vi "XCP DAQ Clear.vi"(8 "error in (no error)":errorcluster, 11 "DAQList in":refnum<class "DAQList.lvclass">) -> (0 "error out":errorcluster, 2 "ECU ref out":T1)   [LabVIEW 2019, in "XCP_DaqDtoId.lvlib" / "DAQList.lvclass"]
uses:
  DAQList.lvclass
  <vilib>/ECUMC/ECUMC.llb/MC Reference.ctt
  DAQList.lvclass/DAQList.ctl
  <vilib>/xnet/xnet.llb/XNET Control Scope.ctl
  <vilib>/ECUMC/ECUMC.lvlib
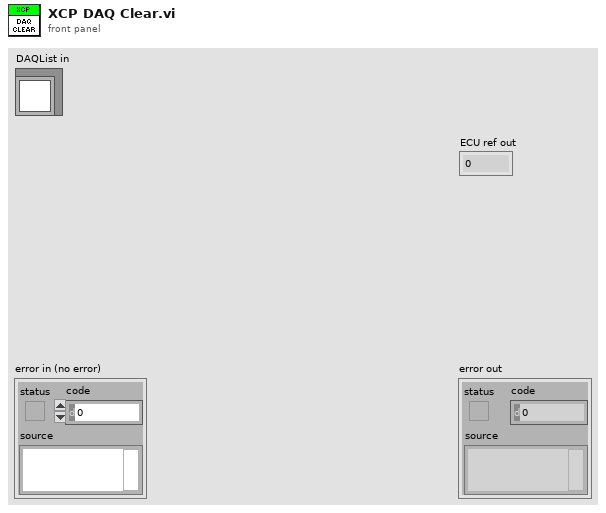
[diagram p1: front panel]
types:
  T1 = typedef "ECUMC.lvlib/MC Reference.ctt" = u32
  T2 = typedef "XNET Control Scope.ctl" = u32
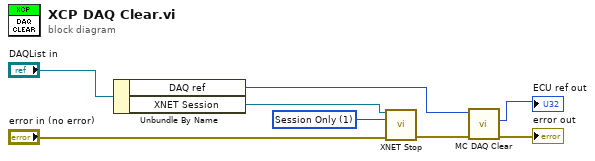
[diagram p0: block diagram]
diagram:
  w3 = T2 1 items=["Normal", "Session Only", "Interface Only", "Session Only Blocking"] ("scope (normal)")
  n1 = Unbundle By Name("DAQList in") -> ("DAQ ref"=w2:T1, "XNET Session"=w4:refnum<k21>)
  n2 = call <vilib>:"XNET Stop.vi"("session in"=w4, "scope (normal)"=w3, "error in (no error)"="error in (no error)") -> ("error out"=w1:errorcluster)  [unwired: 11 in, 1 out]
  n3 = call <vilib>:"MC DAQ Clear.vi"("error in"=w1, "DAQ ref in"=w2) -> ("error out"=→"error out":errorcluster, "ECU ref out"=→"ECU ref out":T1)  [unwired: 8 out]
